vi "search_for_datatype.vi"(1 "control_labels (in)":string[](array[string]), 3 "search_term (in) - i.e. String":string) -> (17 "control_index (-1 = not found)":i32)   [LabVIEW 2016]
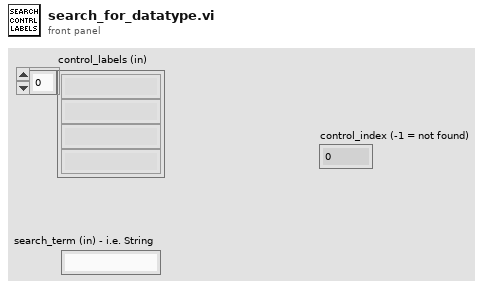
[diagram p1: front panel]
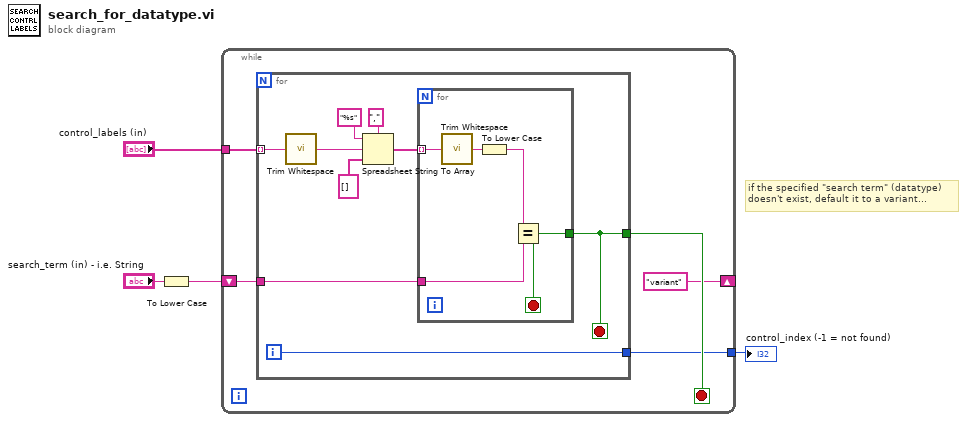
[diagram p0: block diagram]
diagram:
  # "if the specified \"search term\" (datatype)\ndoesn't exist, default it to a variant..."
  n1 = To Lower Case(string="search_term (in) - i.e. String") -> (all lower case string=w2:string)
  n2 = while {
    tunnel: "control_labels (in)" -> [w9]
    shift-right: ["variant"] -> _
    shift-left: w2 -> [w8]
    tunnel: [w5] -> w1
    stop <- w7 stop-if-true
    n3 = for {
      tunnel: w9 -> [w18] mode=indexing
      tunnel: w8 -> [w12]
      tunnel: [w11] -> w7
      tunnel: [w10] -> w5
      i -> [w10]
      stop <- w11 stop-if-true
      n4 = call <vilib>:"Trim Whitespace.vi"("string"=w18) -> ("trimmed string"=w13:string)  [unwired: 1 in]
      n5 = Spreadsheet String To Array(delimiter (Tab)=",", format string="%s", spreadsheet string=w13, array type (2D Dbl)=string[] [] ("control_labels (in)")) -> (array=w14:string[])
      n6 = for {
        tunnel: w14 -> [w23] mode=indexing
        tunnel: w12 -> [w20]
        tunnel: [w19] -> w11
        stop <- w19 stop-if-true
        n7 = call <vilib>:"Trim Whitespace.vi"("string"=w23) -> ("trimmed string"=w22:string)  [unwired: 1 in]
        n8 = To Lower Case(string=w22) -> (all lower case string=w21:string)
        n9 = Equal?(x=w21, y=w20) -> (x = y?=w19:bool)
      }
    }
  }
  "control_index (-1 = not found)" <- w1
